vi "BangBang_GetError.vi"(11 "BANG_BANG":T1 {"Measurment" format="%13.5p"; "Setpoint" format="%13.5p"; "Tolerance" format="%13.5p"}) -> (3 "Error":dbl)   [LabVIEW 2019, in "Trajectory_Library.lvlib"]
doc: "Returns current error, which is Setpoint - Process Variable\n\nInput:\n - BangBang -- Data cluster\n\nOutput:\n - Error -- Current error value."
uses:
  BANG_BANG.ctl
  Trajectory_Library.lvlib
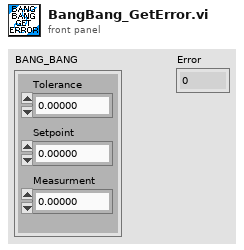
[diagram p1: front panel]
types:
  T1 = typedef "Trajectory_Library.lvlib/BANG_BANG.ctl" = cluster{"Tolerance":dbl, "Setpoint":dbl, "Measurment":dbl}
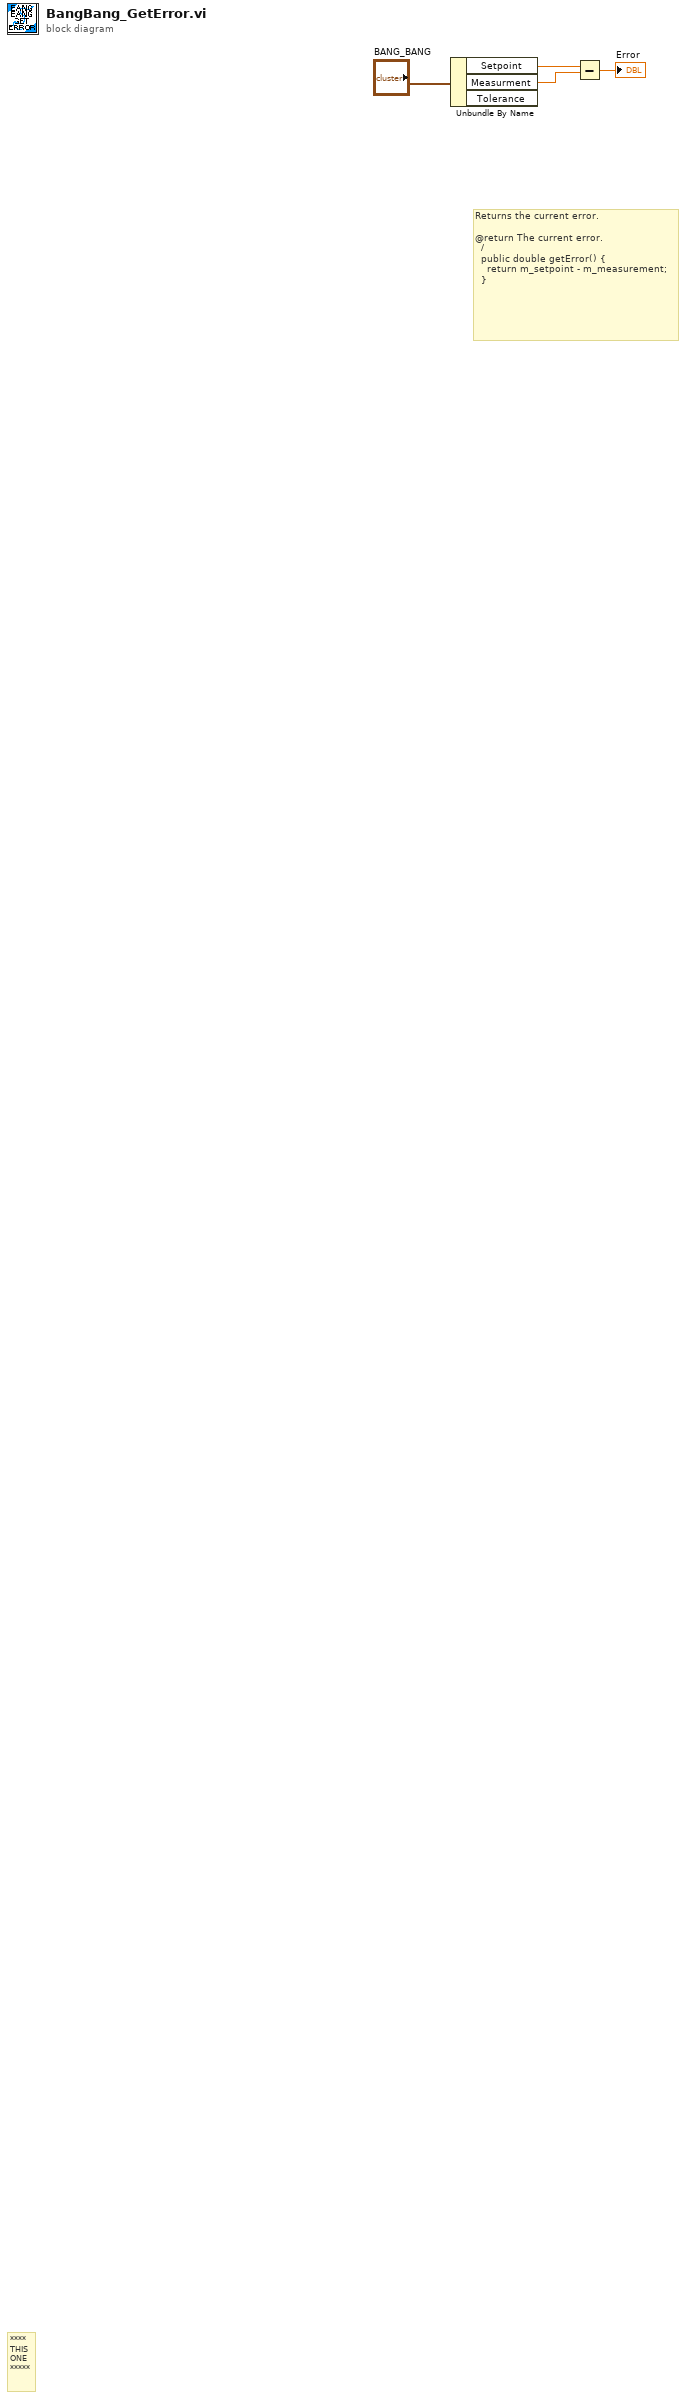
[diagram p0: block diagram]
diagram:
  # "Returns the current error.\n  \n@return The current error.\n  /\n  public double getError() {\n    return m_setpoint - m_measurement;\n  }"
  # "****\nTHIS\nONE\n*****"
  n1 = Unbundle By Name("BANG_BANG") -> ("Setpoint"=w3:dbl, "Measurment"=w2:dbl)  [unwired: 1 out]
  n2 = Subtract(x=w3, y=w2) -> (x-y=→"Error":dbl)
